vi "数据转JSON(子VI).vi"(11 "输出簇":T1) -> (2 "result string":string, 3 "数组":string[](array[string]))   [LabVIEW 2016]
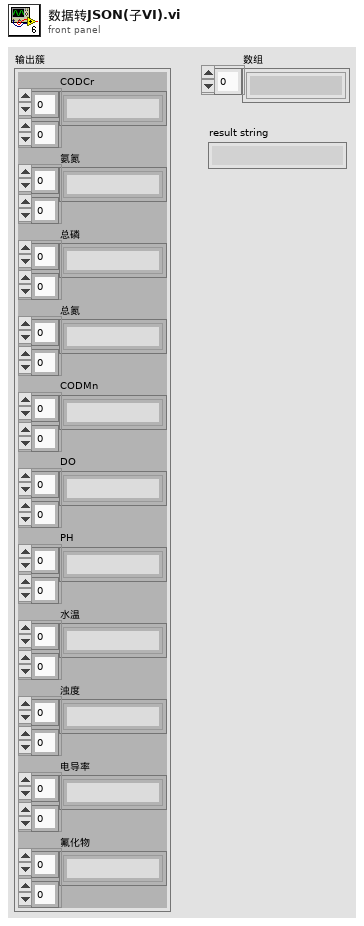
[diagram p1: front panel]
types:
  T1 = cluster{"CODCr":string[][], "氨氮":string[][], "总磷":string[][], "总氮":string[][], "CODMn":string[][], "DO":string[][], "PH":string[][], "水温":string[][], "浊度":string[][], "电导率":string[][], "氟化物":string[][]}
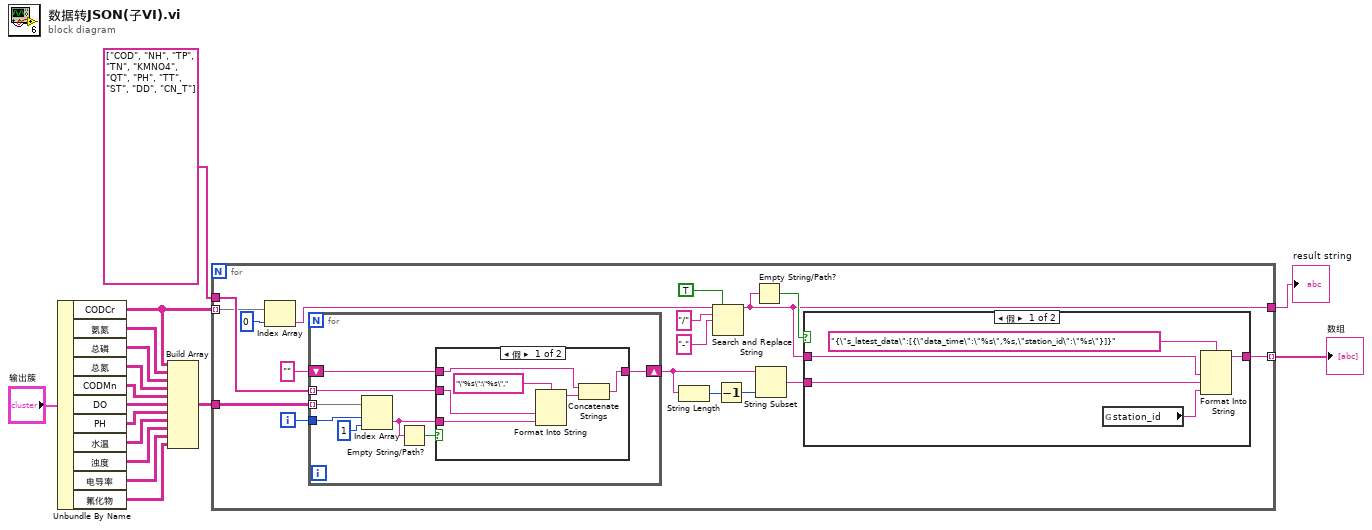
[diagram p0: block diagram]
diagram:
  n1 = Unbundle By Name("输出簇") -> ("CODCr"=w15:string[][], "氨氮"=w3:string[][], "总磷"=w4:string[][], "总氮"=w5:string[][], "CODMn"=w6:string[][], "DO"=w7:string[][], "PH"=w8:string[][], "水温"=w9:string[][], "浊度"=w10:string[][], "电导率"=w11:string[][], "氟化物"=w12:string[][])
  n2 = Build Array(w15, w3, w4, w5, w6, w7, w8, w9, w10, w11, w12) -> (w14:string[][][])
  n3 = for {
    tunnel: string[] ["COD", "NH", "TP", "TN", "KMNO4", "QT", "PH", "TT", "ST", "DD", "CN_T"] -> [w33]
    tunnel: w14 -> [w32]
    tunnel: w15 -> [w31] mode=indexing
    tunnel: [w28] -> w16 mode=indexing
    tunnel: [w17] -> w1
    i -> [w29]
    n4 = Index Array(array=w31, index=0 ("索引")) -> (element=w27:string)
    n5 = for {
      tunnel: w33 -> [w47] mode=indexing
      tunnel: w32 -> [w46] mode=indexing
      tunnel: w29 -> [w43]
      shift-right: [w44] -> w22
      shift-left: "" -> [w40]
      n6 = Index Array(array=w46, index (row)=w43, index (col)=1 ("禁用的索引 (列)")) -> (element=w42:string)
      n7 = Empty String/Path?(string/path=w42) -> (empty?=w41:bool)
      n8 = case shown="假" w41 {
        tunnel: w47 -> [w52 _]
        tunnel: [w48 w54] -> w44
        tunnel: w42 -> [w51 _]
        tunnel: w40 -> [w50 w54]
        frame False {
          n9 = Format Into String(format string="\"%s\":\"%s\"," ("格式字符串"), w52, w51) -> (resulting string=w49:string)  [unwired: 2 in, 1 out]
          n10 = Concatenate Strings(w50, w49) -> (w48:string)
        }
        frame True {
        }
      }
    }
    n11 = String Length(string=w22) -> (length=w21:i32)
    n12 = Search and Replace String(replace all?=TRUE ("替换全部？(F)"), input string=w27, search string="/" ("搜索字符串"), replace string="-" ("替换字符串(\"\")")) -> (result string=w17:string)  [unwired: 4 in, 3 out]
    n13 = Decrement(x=w21) -> (x-1=w20:i32)
    n14 = Empty String/Path?(string/path=w17) -> (empty?=w18:bool)
    n15 = String Subset(string=w22, length (rest)=w20) -> (substring=w19:string)  [unwired: 1 in]
    n16 = case shown="假" w18 {
      tunnel: [w38 w39] -> w28
      tunnel: w19 -> [w37 _]
      tunnel: w17 -> [w36 w39]
      frame False {
        n17 = global read "断电保存全局.vi" "station_id"() -> (w35:string)
        n18 = Format Into String(format string="{\"s_latest_data\":[{\"data_time\":\"%s\",%s,\"station_id\":\"%s\"}]}" ("格式字符串"), w36, w37, w35) -> (resulting string=w38:string)  [unwired: 2 in, 1 out]
      }
      frame True {
      }
    }
  }
  "数组" <- w16
  "result string" <- w1
